vi "AlarmTableChange.vi"(8 "error in (no error)":errorcluster, 10 "AlarmData":string[][](array[string]), 11 "AlarmInfo":refnum<vi>) -> (0 "error out":errorcluster)   [LabVIEW 2017]
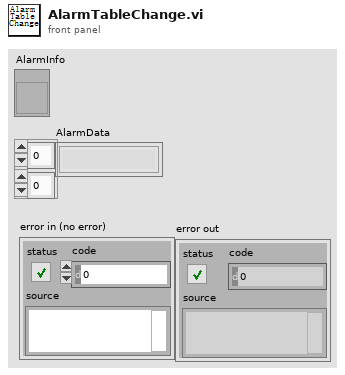
[diagram p1: front panel]
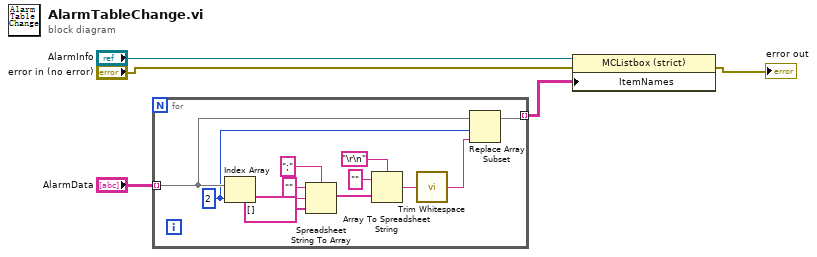
[diagram p0: block diagram]
diagram:
  n1 = for {
    tunnel: "AlarmData" -> [w10] mode=indexing
    tunnel: [w7] -> w3 mode=indexing
    w9 = 2 ("index")
    n2 = Index Array(array=w10, index=w9) -> (element=w17:string)
    n3 = Spreadsheet String To Array(delimiter (Tab)=";", format string="", spreadsheet string=w17, array type (2D Dbl)=string[] []) -> (array=w13:string[])
    n4 = Array To Spreadsheet String(delimiter (Tab)="\r\n", array=w13, 3:"" ("format string")) -> (spreadsheet string=w8:string)
    n5 = call <vilib>:"Trim Whitespace.vi"("string"=w8) -> ("trimmed string"=w6:string)  [unwired: 1 in]
    n6 = Replace Array Subset(array=w10, new element=w6, index=w9) -> (w7:string[])
  }
  n7 = property class="MCListbox (strict)"(reference="AlarmInfo", error in="error in (no error)", "ItemNames"=w3) -> (error out=→"error out":errorcluster)  [unwired: 1 out]
